vi "Get ID Type.vi"(8 "error in (no error)":errorcluster, 11 "id in":refnum<class "id.lvclass">) -> (0 "error out":errorcluster, 2 "type":T1, 3 "id out":refnum<class "id.lvclass">)   [LabVIEW 2016, in "id.lvclass"]
uses:
  id.lvclass
  <vilib>/NI/JSON Support for LabVIEW/JSON Types.ctl
  id.lvclass/id.ctl
  <vilib>/NI/JSON Support for LabVIEW/JSON Data Classes/JSON Datatype/JSON Null.lvclass
  <vilib>/NI/JSON Support for LabVIEW/LVJSON.lvlib
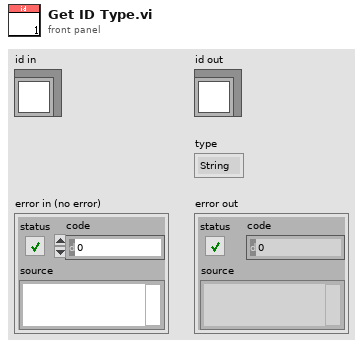
[diagram p1: front panel]
types:
  T1 = typedef "LVJSON.lvlib/JSON Types.ctl" = enum16{"String", "Numeric", "Boolean", "NULL", "Object", "Array"}
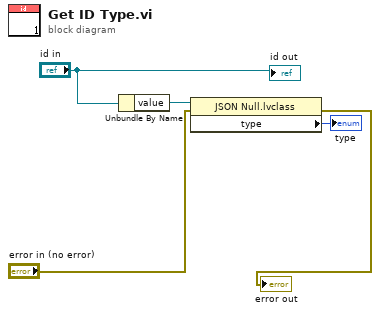
[diagram p0: block diagram]
diagram:
  n1 = Unbundle By Name("id in") -> ("value"=w5:refnum<class "JSON Null.lvclass">)
  n2 = property class="JSON Null.lvclass"(reference=w5, error in="error in (no error)") -> (error out=→"error out":errorcluster, "type"=→"type":T1)  [unwired: 1 out]
  "id out" <- "id in"
